vi "Can Switch Control Types.vi"(9 "Can Switch In":bool, 11 "DAO Actions":T1) -> (1 "Can Switch Out":bool)   [LabVIEW 2009]
uses:
  Data Access Objects/Metadata/DAO Actions.ctl
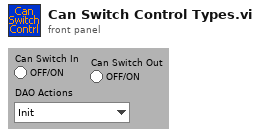
[diagram p1: front panel]
types:
  T1 = typedef "DAO Actions.ctl" = enum16{"Init", "Get", "Set"}
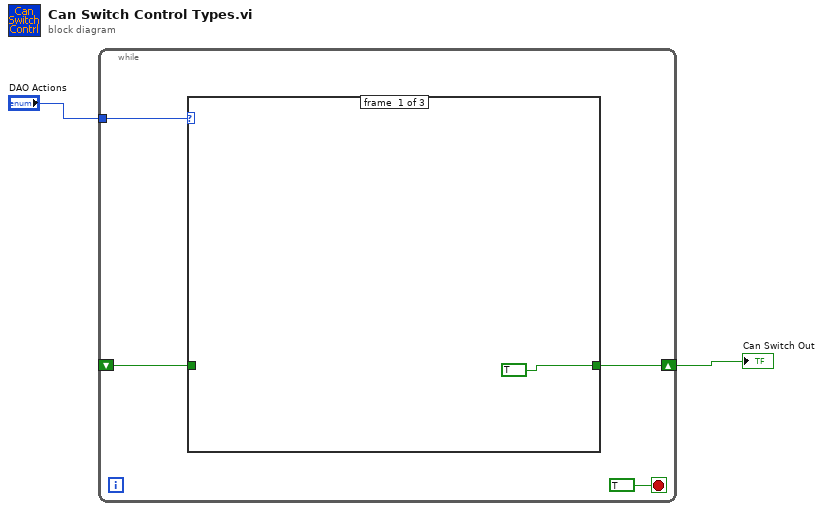
[diagram p0: block diagram]
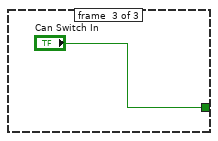
[diagram p3: hidden frame]
diagram:
  n1 = while {
    tunnel: "DAO Actions" -> [w5]
    shift-right: [w4] -> w1
    shift-left: _ -> [w3]
    stop <- TRUE stop-if-true
    n2 = case shown="\"Set\"" w5 {
      tunnel: [TRUE w8 "Can Switch In"] -> w4
      tunnel: w3 -> [_ w8 _]
      frame #0 {
      }
      frame #1 {
      }
      frame #2 {
      }
    }
  }
  "Can Switch Out" <- w1
